vi "FindSphereRim.vi"(0 "number of rim points":i32, 1 "strip (cm)":cluster{"radius":dbl, "h":dbl, "w":dbl} {"w" format="%.2f"; "h" format="%.2f"; "radius" format="%.2f"}) -> (2 "x":dbl[](array[numeric]) format="%.2f", 3 "y":dbl[](array[numeric]) format="%.2f", 4 "z":dbl[](array[numeric]) format="%.2f", 5 "d":dbl format="%.2f")   [LabVIEW 2022 SP3]
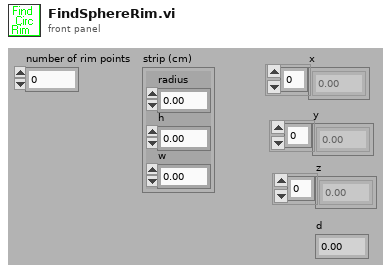
[diagram p1: front panel]
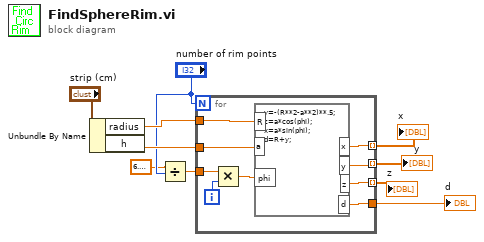
[diagram p0: block diagram]
diagram:
  n1 = Unbundle By Name("strip (cm)") -> ("radius"=w8:dbl, "h"=w9:dbl)
  n2 = Divide(x=6.283185307179586, y="number of rim points") -> (x/y=w5:dbl)
  n3 = for {
    N: "number of rim points" -> [_]
    tunnel: [w19] -> w2 mode=indexing
    tunnel: w5 -> [w18]
    tunnel: w9 -> [w15]
    tunnel: [w14] -> w3 mode=indexing
    tunnel: [w13] -> w1 mode=indexing
    tunnel: w8 -> [w12]
    tunnel: [w11] -> w10
    i -> [w17]
    n4 = Multiply(x=w18, y=w17) -> (x*y=w16:dbl)
    n5 = formula code="y=-(R**2-a**2)**.5;\nz=a*cos(phi);\nx=a*sin(phi);\nd=R+y;"("phi"=w16, "R"=w12, "a"=w15) -> ("x"=w14:dbl, "z"=w13:dbl, "y"=w19:dbl, "d"=w11:dbl)
  }
  "d" <- w10
  "z" <- w1
  "y" <- w2
  "x" <- w3
